vi "Populate Copy.vi"(8 "error in (no error)":errorcluster, 10 "Msg to Populate":refnum<class "Response Msg.lvclass">, 11 "Source Msg":refnum<class "Flex Msg.lvclass">) -> (0 "error out":errorcluster, 2 "Populated Msg":refnum<class "Response Msg.lvclass">)   [LabVIEW 2020, in "Publisher.lvlib" / "Response Msg.lvclass"]
doc: "Populate 'Msg to Populate' with data from 'Source Msg'. Use this VI if some private data is required for the operation of the message and cannot be written in any other way (as in nested message execution).\n\nThis implementation transfers the Core and 'Sender is Waiting?', not 'Publish?'."
uses:
  Response Msg.lvclass
  C:/Current projects/WS/PPL/HDH.Actor Framework.Core.Msg.lvlibp/Flex Msg/Flex Msg.lvclass
  PPL/HDH.Actor Framework.Core.Msg.lvlibp/Flex Msg/Flex Msg.lvclass
  Response Msg.lvclass/Response Msg.ctl
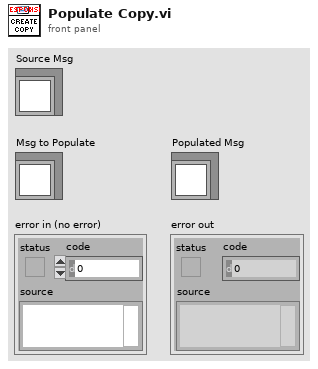
[diagram p1: front panel]
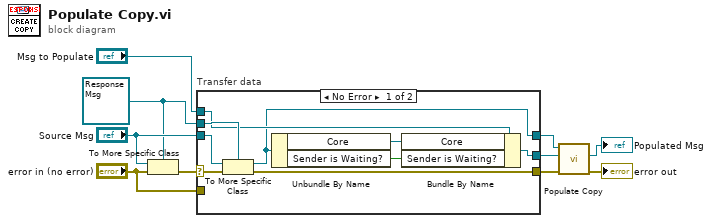
[diagram p0: block diagram]
diagram:
  w5 = refnum<class "Response Msg.lvclass"> refnum ("Msg to Populate 2")
  n1 = To More Specific Class(target class=w5, reference="Source Msg", error in="error in (no error)") -> (error out=w8:errorcluster)  [unwired: 1 out]
  n2 = case "Transfer data" shown="No Error" w8 {
    selector: w8 -> [w19 _]
    tunnel: [w12 w22] -> w6
    tunnel: "Source Msg" -> [w18 w22]
    tunnel: w5 -> [w17 _]
    tunnel: "Msg to Populate" -> [w16 w21]
    tunnel: [w15 w21] -> w3
    tunnel: [w11 w20] -> w2
    tunnel: "error in (no error)" -> [_ w20]
    frame No Error {
      n3 = To More Specific Class(target class=w17, reference=w18, error in=w19) -> (specific class reference=w12:refnum<class "Response Msg.lvclass">, error out=w11:errorcluster)
      n4 = Unbundle By Name(w12) -> ("Core"=w14:refnum<class "Response Core.lvclass">, "Sender is Waiting?"=w13:bool)
      n5 = Bundle By Name(cluster=w16, "Core"=w14, "Sender is Waiting?"=w13) -> (w15:refnum<class "Response Msg.lvclass">)
    }
    frame Error {
    }
  }
  n6 = call-parent "Populate Copy.vi"("error in (no error)"=w2, "Msg to Populate"=w3, "Source Msg"=w6) -> ("error out"=→"error out":errorcluster, "Populated Msg"=→"Populated Msg":refnum<class "Response Msg.lvclass">)  [unwired: 7 in]
